vi "test Decode Parameters for Labels in a Channel.vi"(8 "error in":errorcluster, 11 "TestCase in":refnum<class "Engine.lvclass">) -> (0 "error out":errorcluster, 3 "TestCase out":refnum<class "Engine.lvclass">)   [LabVIEW 2020, in "Engine.lvclass"]
uses:
  Engine.lvclass
  Shared/RT Label Settings.ctl
  Shared/Label.ctl
  Shared/RT Parameters.ctl
  Shared/Parameter Definition.ctl
  <vilib>/NI/NI VeriStand Encoding and Decoding/Encoding.ctl
  <vilib>/NI VeriStand/Custom Device API/Custom Device Item Ref.ctl
  Shared/Transfer Type.ctl
  <vilib>/NI VeriStand/Custom Device API/Data Reference.ctl
  <vilib>/addons/_JKI Toolkits/VI Tester/TestCase.llb/TestCase.lvclass
  Engine/Implementation/Rx Execution Unit/Rx Execution Unit.lvclass
  <vilib>/NI VeriStand/Custom Device API/Custom Device API.lvlib
  <vilib>/NI/NI VeriStand Encoding and Decoding/Encoding and Decoding.lvlib
  C:/Program Files (x86)/National Instruments/LabVIEW 2020/vi.lib/addons/_JKI Toolkits/VI Tester/TestCase.llb/TestCase.lvclass
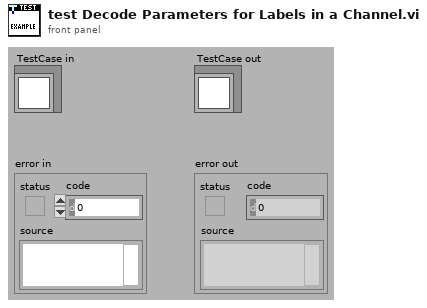
[diagram p1: front panel]
types:
  T1 = typedef "RT Label Settings.ctl" = cluster{"Name":string, "xmlName":string, "label":T2, "transfer period":u32, "SDI_Enabled":bool, "SDI":u8, "parameter driver data":T3, "transfer type":T7, "has timestamp?":bool, "Label Disable/Trigger Channel Reference":T6, "Message Handle":u64, "Initialized?":bool, "Word Initial Raw Value":u32, "Label Timestamp Channel Data Reference":T8, "disabled":bool}
  T2 = typedef "Label.ctl" = u8
  T3 = typedef "RT Parameters.ctl" = cluster{"parameter definitions":T4[], "Tx parameter refs":T6[]}
  T4 = typedef "Parameter Definition.ctl" = cluster{"start index":i32, "size":i32, "encoding":T5, "signed":bool, "scale multiplier":dbl, "scale offset":dbl, "default value":dbl}
  T5 = typedef "Encoding and Decoding.lvlib/Encoding.ctl" = enum16{"BNR", "BCD", "Discrete"}
  T6 = typedef "Custom Device API.lvlib/Custom Device Item Ref.ctl" = u64
  T7 = typedef "Transfer Type.ctl" = enum16{"Scheduled", "Acyclic", "Block", "Strobe"}
  T8 = typedef "Custom Device API.lvlib/Data Reference.ctl" = i32
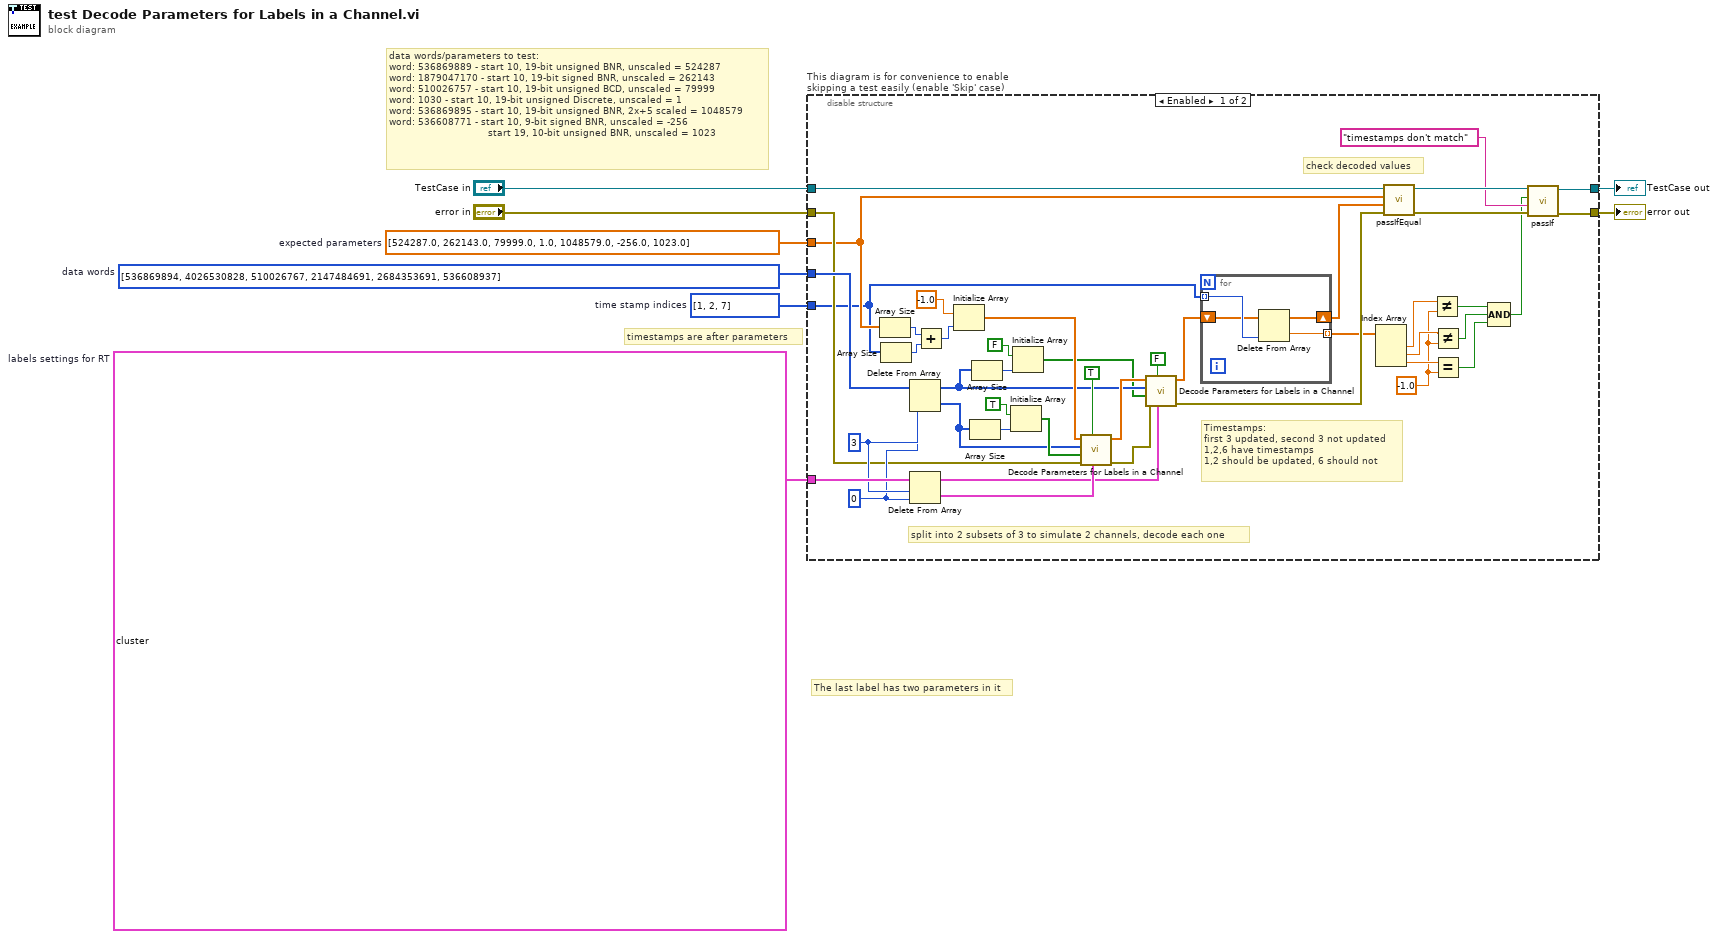
[diagram p0: block diagram]
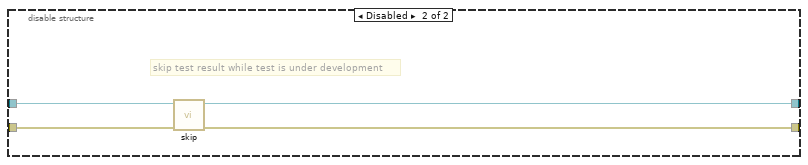
[diagram p2: hidden frame]
diagram:
  w1 = i32[] [1, 2, 7]  # time stamp indices
  w3 = dbl[] [524287.0, 262143.0, 79999.0, 1.0, 1048579.0, -256.0, 1023.0]  # expected parameters
  w4 = T1[] [{"Name"="", "xmlName"="", "label"=0, "transfer period"=0, "SDI_Enabled"=FALSE, "SDI"=0, "parameter driver data"={"parameter definitions"=[{"start index"=10, "size"=19, "encoding"=enum."BNR", "signed"=FALSE, "scale multiplier"=1.0, "scale offset"=0.0, "default value"=0.0}], "Tx parameter refs"=[]}, "transfer type"=enum."Scheduled", "has timestamp?"=TRUE, "Label Disable/Trigger Channel Reference"=0, "Message Handle"=0, "Initialized?"=FALSE, "Word Initial Raw Value"=0, "Label Timestamp Channel Data Reference"=0, "disabled"=FALSE}, {"Name"="", "xmlName"="", "label"=0, "transfer period"=0, "SDI_Enabled"=FALSE, "SDI"=0, "parameter driver data"={"parameter definitions"=[{"start index"=10, "size"=19, "encoding"=enum."BNR", "signed"=TRUE, "scale multiplier"=1.0, "scale offset"=0.0, "default value"=0.0}], "Tx parameter refs"=[]}, "transfer type"=enum."Scheduled", "has timestamp?"=TRUE, "Label Disable/Trigger Channel Reference"=0, "Message Handle"=0, "Initialized?"=FALSE, "Word Initial Raw Value"=0, "Label Timestamp Channel Data Reference"=0, "disabled"=FALSE}, {"Name"="", "xmlName"="", "label"=0, "transfer period"=0, "SDI_Enabled"=FALSE, "SDI"=0, "parameter driver data"={"parameter definitions"=[{"start index"=10, "size"=19, "encoding"=enum."BCD", "signed"=FALSE, "scale multiplier"=1.0, "scale offset"=0.0, "default value"=0.0}], "Tx parameter refs"=[]}, "transfer type"=enum."Scheduled", "has timestamp?"=FALSE, "Label Disable/Trigger Channel Reference"=0, "Message Handle"=0, "Initialized?"=FALSE, "Word Initial Raw Value"=0, "Label Timestamp Channel Data Reference"=0, "disabled"=FALSE}, {"Name"="", "xmlName"="", "label"=0, "transfer period"=0, "SDI_Enabled"=FALSE, "SDI"=0, "parameter driver data"={"parameter definitions"=[{"start index"=10, "size"=19, "encoding"=enum."Discrete", "signed"=FALSE, "scale multiplier"=1.0, "scale offset"=0.0, "default value"=0.0}], "Tx parameter refs"=[]}, "transfer type"=enum."Scheduled", "has timestamp?"=FALSE, "Label Disable/Trigger Channel Reference"=0, "Message Handle"=0, "Initialized?"=FALSE, "Word Initial Raw Value"=0, "Label Timestamp Channel Data Reference"=0, "disabled"=FALSE}, {"Name"="", "xmlName"="", "label"=0, "transfer period"=0, "SDI_Enabled"=FALSE, "SDI"=0, "parameter driver data"={"parameter definitions"=[{"start index"=10, "size"=19, "encoding"=enum."BNR", "signed"=FALSE, "scale multiplier"=2.0, "scale offset"=5.0, "default value"=0.0}], "Tx parameter refs"=[]}, "transfer type"=enum."Scheduled", "has timestamp?"=FALSE, "Label Disable/Trigger Channel Reference"=0, "Message Handle"=0, "Initialized?"=FALSE, "Word Initial Raw Value"=0, "Label Timestamp Channel Data Reference"=0, "disabled"=FALSE}, {"Name"="", "xmlName"="", "label"=0, "transfer period"=0, "SDI_Enabled"=FALSE, "SDI"=0, "parameter driver data"={"parameter definitions"=[{"start index"=10, "size"=9, "encoding"=enum."BNR", "signed"=TRUE, "scale multiplier"=1.0, "scale offset"=0.0, "default value"=0.0}, {"start index"=19, "size"=10, "encoding"=enum."BNR", "signed"=FALSE, "scale multiplier"=1.0, "scale offset"=0.0, "default value"=0.0}], "Tx parameter refs"=[]}, "transfer type"=enum."Scheduled", "has timestamp?"=TRUE, "Label Disable/Trigger Channel Reference"=0, "Message Handle"=0, "Initialized?"=FALSE, "Word Initial Raw Value"=0, "Label Timestamp Channel Data Reference"=0, "disabled"=FALSE}]  # labels settings for RT
  w5 = u32[] [536869894, 4026530828, 510026767, 2147484691, 2684353691, 536608937]  # data words
  # "timestamps are after parameters"
  # "The last label has two parameters in it"
  # "for visibility, irrelevant label settings are minimized in this constant"
  # "data words/parameters to test:\nword: 536869889 - start 10, 19-bit unsigned BNR, unscaled = 524287\nword: 1879047170 - start 10, 19-bit signed BNR, unscaled = 262143\nword: 510026757 - start 10, 19-bit unsigned BCD, unscaled = 79999\nword: 1030 - start 10, 19-bit unsigned Discrete, unscaled = 1\nword: 536869895 - start 10, 19-bit unsigned BNR, 2x+5 scaled = 1048579 \nword: 536608771 - start 10, 9-bit signed BNR, unscaled = -256\n                                 start 19, 10-bit unsigned BNR, unscaled = 1023"
  n1 = disable-structure "This diagram is for convenience to enable skipping a test easily (enable 'Skip' case)" shown="Enabled" {
    disable-tunnel: "TestCase in" -> [w50 w60]
    disable-tunnel: [w23 w58] -> w2
    disable-tunnel: [w25 w59] -> w7
    disable-tunnel: "error in" -> [w46 w57]
    disable-tunnel: w5 -> [w51 _]
    disable-tunnel: w4 -> [w52 _]
    disable-tunnel: w3 -> [w42 _]
    disable-tunnel: w1 -> [w20 _]
    frame Enabled {
      w13 = -1.0
      w48 = 0 ("index")
      w49 = 3 ("length")
      # "Timestamps: \nfirst 3 updated, second 3 not updated\n1,2,6 have timestamps\n1,2 should be updated, 6 should not"
      # "check decoded values"
      # "split into 2 subsets of 3 to simulate 2 channels, decode each one"
      n2 = Array Size(array=w42) -> (size(s)=w18:i32)
      n3 = Array Size(array=w20) -> (size(s)=w19:i32)
      n4 = Delete From Array(array=w51, length=w49, index=w48) -> (deleted portion=w29:u32[], array with subset deleted=w36:u32[])
      n5 = Delete From Array(array=w52, length=w49, index=w48) -> (deleted portion=w38:T1[], array with subset deleted=w37:T1[])
      n6 = Add(x=w18, y=w19) -> (x+y=w17:i32)
      n7 = Initialize Array(-1.0 ("element"), w17) -> (w43:dbl[])
      n8 = Array Size(array=w29) -> (size(s)=w31:i32)
      n9 = Array Size(array=w36) -> (size(s)=w35:i32)
      n10 = Initialize Array(TRUE, w31) -> (w30:bool[])
      n11 = Initialize Array(FALSE, w35) -> (w33:bool[])
      n12 = call "Decode Parameters for Labels in a Channel.vi"("labels settings for RT"=w38, "reset index"=TRUE, "error in (no error)"=w46, "updated labels?"=w30, "data words in"=w29, "Parameter Values in"=w43) -> ("error out"=w45:errorcluster, "Parameter Values out"=w41:dbl[])  [unwired: 4 in]
      n13 = call "Decode Parameters for Labels in a Channel.vi"("labels settings for RT"=w37, "reset index"=FALSE, "error in (no error)"=w45, "updated labels?"=w33, "data words in"=w36, "Parameter Values in"=w41) -> ("error out"=w47:errorcluster, "Parameter Values out"=w28:dbl[])  [unwired: 4 in]
      n14 = for {
        tunnel: w20 -> [w56] mode=indexing
        shift-right: [w54] -> w21
        shift-left: w28 -> [w55]
        tunnel: [w53] -> w27 mode=indexing
        n15 = Delete From Array(array=w55, index=w56) -> (deleted portion=w53:dbl, array with subset deleted=w54:dbl[])  [unwired: 1 in]
      }
      n16 = Index Array(array=w27) -> (element #1=w16:dbl, element #2=w15:dbl, element #3=w14:dbl)  [unwired: 3 in]
      n17 = call-dynamic "passIfEqual.vi"("error in (no error)"=w47, "y"=w21, "x"=w42, "TestCase in"=w50) -> ("error out"=w26:errorcluster, "TestCase out"=w24:refnum<class "Engine.lvclass">)  [unwired: 6 in]
      n18 = Not Equal?(x=w16, y=w13) -> (x != y?=w12:bool)
      n19 = Not Equal?(x=w15, y=w13) -> (x != y?=w11:bool)
      n20 = Equal?(x=w14, y=w13) -> (x = y?=w10:bool)
      n21 = Compound Arithmetic op=AND(w12, w11, w10) -> (w9:bool)
      n22 = call-dynamic "passIf.vi"("error in (no error)"=w26, "message (\"\")"="timestamps don't match" ("message (\"\")"), "pass"=w9, "TestCase in"=w24) -> ("error out"=w25:errorcluster, "TestCase out"=w23:refnum<class "Engine.lvclass">)  [unwired: 6 in]
    }
    frame Disabled {
      # "skip test result while test is under development"
      n23 = call <vilib>:"skip.vi"("error in (no error)"=w57, "TestCase in"=w60) -> ("error out"=w59:errorcluster, "TestCase out"=w58:refnum<class "Engine.lvclass">)  [unwired: 8 in]
    }
  }
  "error out" <- w7
  "TestCase out" <- w2
